vi "M686_Init.vi"() -> (1 "Status":bool, 2 "Positions":dbl[](array[numeric]), 3 "VISA Refnum out":refnum<visa-resource-name>)   [LabVIEW 2014]
uses:
  <vilib>/Instr/_visa.llb/VISA Configure Serial Port (Instr).vi
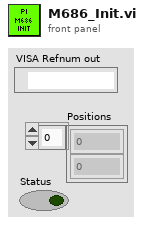
[diagram p1: front panel]
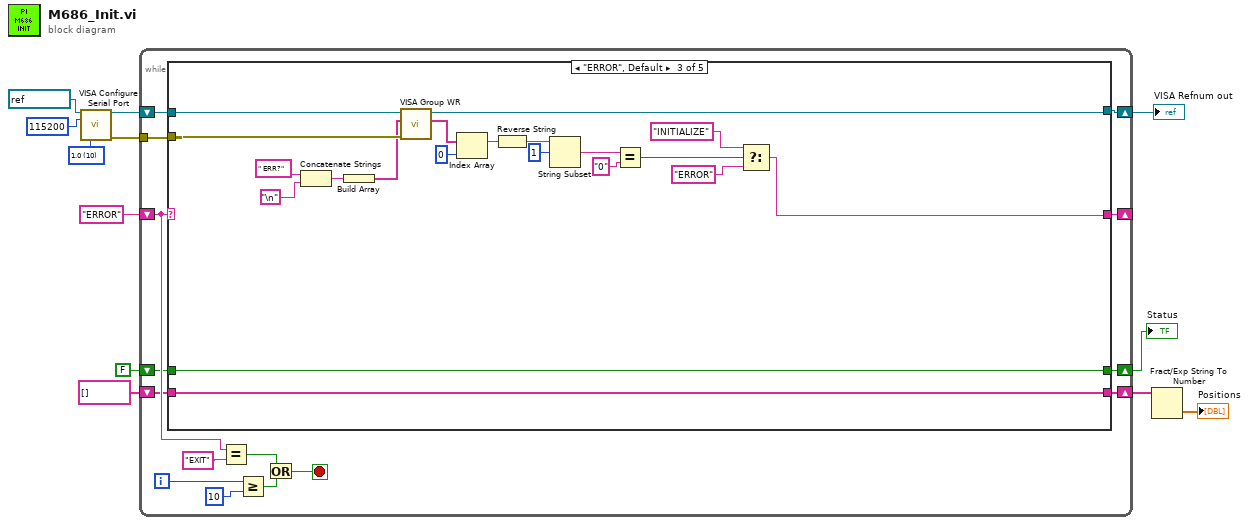
[diagram p0: block diagram]
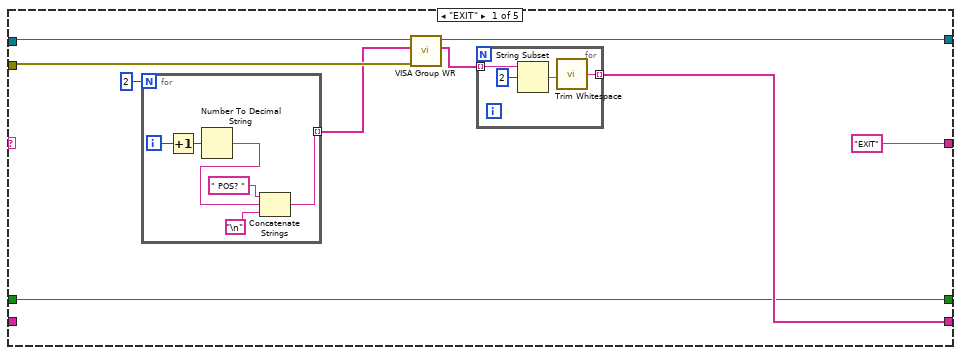
[diagram p2: hidden frame]
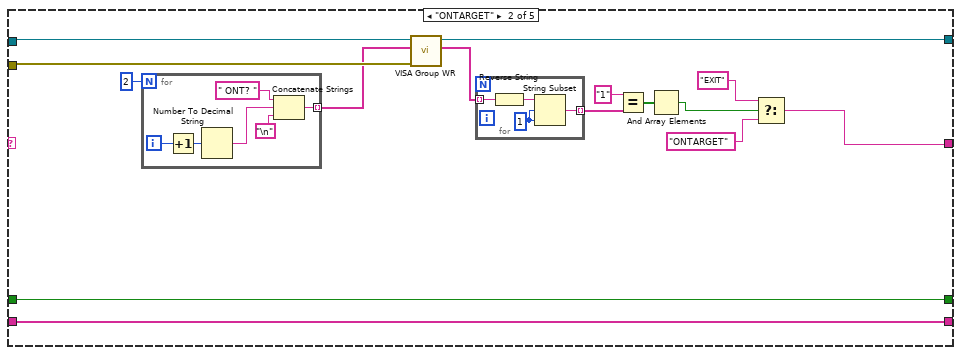
[diagram p3: hidden frame]
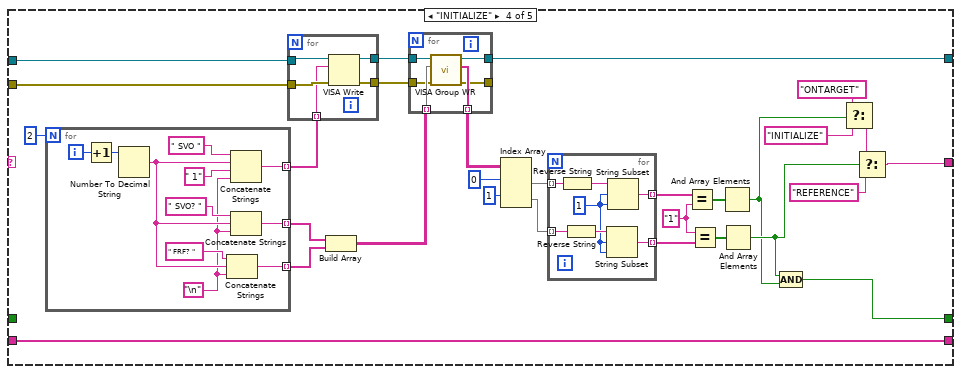
[diagram p4: hidden frame]
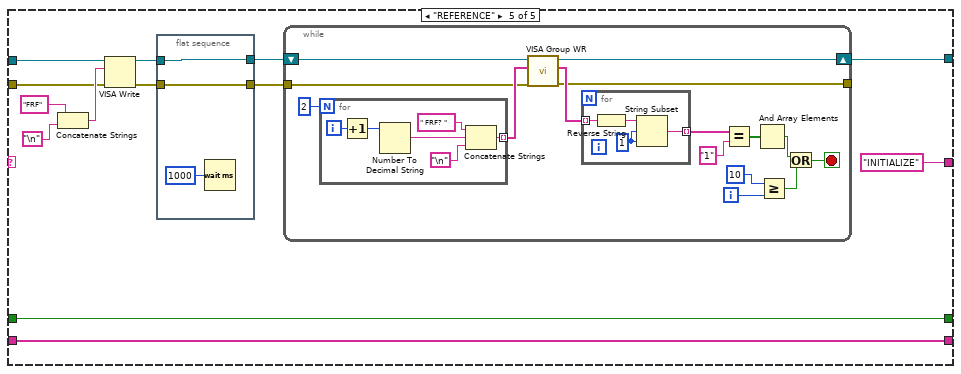
[diagram p5: hidden frame]
diagram:
  w8 = u16 10 items=["1.0"=10, "1.5"=15, "2.0"=20] ("stop bits (10: 1 bit)")
  n1 = call-poly "VISA Configure Serial Port"("VISA resource name"=refnum<visa-resource-name> "COM7", "baud rate (9600)"=u32 115200, "stop bits (10: 1 bit)"=w8) -> ("VISA resource name out"=w12:refnum<visa-resource-name>, "error out"=w9:errorcluster)  [unwired: 11 in]
  n2 = while {
    tunnel: w9 -> [w26]
    shift-right: [w25] -> _
    shift-left: "ERROR" -> [w23]
    shift-right: [w15] -> w5
    shift-left: w12 -> [w27]
    shift-right: [w16] -> w2
    shift-left: string[] [] -> [w14]
    shift-right: [w19] -> w11
    shift-left: FALSE -> [w13]
    i -> [w17]
    stop <- w21 stop-if-true
    n3 = case shown="\"ERROR\", Default" w23 {
      tunnel: w27 -> [w35 w61 w89 w117 w159]
      tunnel: w26 -> [w34 w60 w88 w116 w158]
      tunnel: [w28 w48 w73 w96 w155] -> w19
      tunnel: ["EXIT" w49 w74 w102 "INITIALIZE"] -> w25
      tunnel: [w30 w47 w72 w92 w154] -> w16
      tunnel: [w29 w57 w79 w93 w156] -> w15
      tunnel: w14 -> [_ w47 w72 w92 w154]
      tunnel: w13 -> [w28 w48 w73 _ w155]
      frame "EXIT" {
        n4 = for {
          N: 2 -> [_]
          tunnel: [w46] -> w32 mode=indexing
          i -> [w43]
          n5 = Increment(x=w43) -> (x+1=w44:i32)
          n6 = Number To Decimal String(number=w44) -> (decimal integer string=w41:string)  [unwired: 1 in]
          n7 = Concatenate Strings(" POS? " ("string"), w41, "\n") -> (w46:string)
        }
        n8 = call "VISA Group WR.vi"("error in (no error)"=w34, "Array in"=w32, "VISA Refnum in"=w35) -> ("Array out"=w31:string[], "VISA Refnum out"=w29:refnum<visa-resource-name>)  [unwired: 6 in, 1 out]
        n9 = for {
          tunnel: w31 -> [w40] mode=indexing
          tunnel: [w37] -> w30 mode=indexing
          n10 = String Subset(string=w40, offset (0)=2) -> (substring=w38:string)  [unwired: 1 in]
          n11 = call <vilib>:"Trim Whitespace.vi"("string"=w38) -> ("trimmed string"=w37:string)  [unwired: 1 in]
        }
      }
      frame "ONTARGET" {
        n12 = for {
          N: 2 -> [_]
          tunnel: [w71] -> w58 mode=indexing
          i -> [w68]
          n13 = Increment(x=w68) -> (x+1=w69:i32)
          n14 = Number To Decimal String(number=w69) -> (decimal integer string=w66:string)  [unwired: 1 in]
          n15 = Concatenate Strings(" ONT? " ("string"), w66, "\n") -> (w71:string)
        }
        n16 = call "VISA Group WR.vi"("error in (no error)"=w60, "Array in"=w58, "VISA Refnum in"=w61) -> ("Array out"=w54:string[], "VISA Refnum out"=w57:refnum<visa-resource-name>)  [unwired: 6 in, 1 out]
        n17 = for {
          tunnel: [w62] -> _ mode=indexing
          tunnel: [w63] -> w55 mode=indexing
          tunnel: w54 -> [w62] mode=indexing
          w64 = 1 ("length (rest)")
          n18 = Reverse String(1:w62) -> (0:w65:string)
          n19 = String Subset(string=w65, offset (0)=w64, length (rest)=w64) -> (substring=w63:string)
        }
        n20 = Equal?(x="1", y=w55) -> (x = y?=w56:bool[])
        n21 = And Array Elements(Boolean array=w56) -> (logical AND=w52:bool)
        n22 = Select(t="EXIT", s=w52, f="ONTARGET") -> (s? t:f=w49:string)
      }
      frame "ERROR", Default {
        n23 = Concatenate Strings(" ERR?" ("string"), "\n") -> (w87:string)
        n24 = Build Array(w87) -> (w86:string[])
        n25 = call "VISA Group WR.vi"("error in (no error)"=w88, "Array in"=w86, "VISA Refnum in"=w89) -> ("Array out"=w82:string[], "VISA Refnum out"=w79:refnum<visa-resource-name>)  [unwired: 6 in, 1 out]
        n26 = Index Array(array=w82, index=0) -> (element=w81:string)
        n27 = Reverse String(1:w81) -> (0:w83:string)
        n28 = String Subset(string=w83, offset (0)=1) -> (substring=w85:string)  [unwired: 1 in]
        n29 = Equal?(x=w85, y="0") -> (x = y?=w77:bool)
        n30 = Select(t="INITIALIZE", s=w77, f="ERROR") -> (s? t:f=w74:string)
      }
      frame "INITIALIZE" {
        w100 = "1"
        n31 = for {
          N: 2 -> [_]
          tunnel: [w149] -> w115 mode=indexing
          tunnel: [w148] -> w114 mode=indexing
          tunnel: [w147] -> w113 mode=indexing
          i -> [w145]
          w139 = "\n"
          n32 = Increment(x=w145) -> (x+1=w146:i32)
          n33 = Number To Decimal String(number=w146) -> (decimal integer string=w141:string)  [unwired: 1 in]
          n34 = Concatenate Strings(" FRF? " ("string"), w141, w139) -> (w147:string)
          n35 = Concatenate Strings(" SVO " ("string"), w141, " 1" ("string"), w139) -> (w149:string)
          n36 = Concatenate Strings(" SVO? " ("string"), w141, w139) -> (w148:string)
        }
        n37 = for {
          tunnel: w117 -> [w138]
          tunnel: w116 -> [w137]
          tunnel: [w136] -> w118
          tunnel: [w135] -> w119
          tunnel: w115 -> [w134] mode=indexing
          n38 = VISA Write(VISA resource name=w138, write buffer=w134, error in (no error)=w137) -> (VISA resource name out=w136:refnum<visa-resource-name>, error out=w135:errorcluster)  [unwired: 1 out]
        }
        n39 = Build Array(w114, w113) -> (w112:string[][])
        n40 = for {
          tunnel: w118 -> [w133]
          tunnel: w112 -> [w132] mode=indexing
          tunnel: [w131] -> w103 mode=indexing
          tunnel: [w130] -> w93
          tunnel: w119 -> [w129]
          tunnel: [w128] -> _
          n41 = call "VISA Group WR.vi"("error in (no error)"=w129, "Array in"=w132, "VISA Refnum in"=w133) -> ("error out"=w128:errorcluster, "Array out"=w131:string[], "VISA Refnum out"=w130:refnum<visa-resource-name>)  [unwired: 6 in]
        }
        n42 = Index Array(array=w103, index (row) #1=0 ("index (row)"), index (row) #2=1 ("index (row)")) -> (element #1=w107:string[], element #2=w108:string[])  [unwired: 2 in]
        n43 = for {
          tunnel: w107 -> [w126] mode=indexing
          tunnel: [w125] -> w110 mode=indexing
          tunnel: w108 -> [w123] mode=indexing
          tunnel: [w122] -> w101 mode=indexing
          w121 = 1 ("length (rest)")
          n44 = Reverse String(1:w126) -> (0:w127:string)
          n45 = Reverse String(1:w123) -> (0:w124:string)
          n46 = String Subset(string=w124, offset (0)=w121, length (rest)=w121) -> (substring=w122:string)
          n47 = String Subset(string=w127, offset (0)=w121, length (rest)=w121) -> (substring=w125:string)
        }
        n48 = Equal?(x=w110, y=w100) -> (x = y?=w109:bool[])
        n49 = Equal?(x=w100, y=w101) -> (x = y?=w106:bool[])
        n50 = And Array Elements(Boolean array=w109) -> (logical AND=w94:bool)
        n51 = And Array Elements(Boolean array=w106) -> (logical AND=w95:bool)
        n52 = Compound Arithmetic op=AND(w95, w94) -> (w96:bool)
        n53 = Select(t="ONTARGET", s=w94, f="INITIALIZE") -> (s? t:f=w97:string)
        n54 = Select(t=w97, s=w95, f="REFERENCE") -> (s? t:f=w102:string)
      }
      frame "REFERENCE" {
        n55 = Concatenate Strings("FRF" ("string"), "\n") -> (w160:string)
        n56 = VISA Write(VISA resource name=w159, write buffer=w160, error in (no error)=w158) -> (VISA resource name out=w152:refnum<visa-resource-name>, error out=w150:errorcluster)  [unwired: 1 out]
        n57 = flat-sequence {
          tunnel: [w165] -> w153
          tunnel: w152 -> [w165]
          tunnel: [w164] -> w151
          tunnel: w150 -> [w164]
          frame #0 {
            n58 = Wait (ms)(milliseconds to wait=u32 1000) -> ()  [unwired: 1 out]
          }
        }
        n59 = while {
          tunnel: w151 -> [w172]
          tunnel: [w171] -> _
          shift-right: [w179] -> w156
          shift-left: w153 -> [w180]
          i -> [w169]
          stop <- w167 stop-if-true
          n60 = for {
            N: 2 -> [_]
            tunnel: [w190] -> w178 mode=indexing
            i -> [w187]
            n61 = Increment(x=w187) -> (x+1=w189:i32)
            n62 = Number To Decimal String(number=w189) -> (decimal integer string=w186:string)  [unwired: 1 in]
            n63 = Concatenate Strings(" FRF? " ("string"), w186, "\n") -> (w190:string)
          }
          n64 = call "VISA Group WR.vi"("error in (no error)"=w172, "Array in"=w178, "VISA Refnum in"=w180) -> ("error out"=w171:errorcluster, "Array out"=w177:string[], "VISA Refnum out"=w179:refnum<visa-resource-name>)  [unwired: 6 in]
          n65 = for {
            tunnel: w177 -> [w182] mode=indexing
            tunnel: [w181] -> w174 mode=indexing
            w184 = 1 ("length (rest)")
            n66 = Reverse String(1:w182) -> (0:w183:string)
            n67 = String Subset(string=w183, offset (0)=w184, length (rest)=w184) -> (substring=w181:string)
          }
          n68 = Equal?(x=w174, y="1") -> (x = y?=w175:bool[])
          n69 = And Array Elements(Boolean array=w175) -> (logical AND=w173:bool)
          n70 = Greater Or Equal?(x=10, y=w169) -> (x >= y?=w166:bool)
          n71 = Or(x=w173, y=w166) -> (x .or. y?=w167:bool)
        }
      }
    }
    n72 = Equal?(x=w23, y="EXIT") -> (x = y?=w22:bool)
    n73 = Greater Or Equal?(x=w17, y=10 ("x")) -> (x >= y?=w20:bool)
    n74 = Or(x=w22, y=w20) -> (x .or. y?=w21:bool)
  }
  "VISA Refnum out" <- w5
  "Status" <- w11
  n75 = Fract/Exp String To Number(string=w2) -> (number=→"Positions":dbl[])  [unwired: 3 in, 1 out]
